vi "Example Write Read Type 2 - StateChanged Callback.vi"(4 "StateChanged":refnum<user-event>, 5 "Event Data":T1, 6 "Control Ref":refnum<k24>, 7 "Event Common Data":T2) -> ()   [LabVIEW 2010]
uses:
  C:/tf/play/labview/Tinkerforge.dll
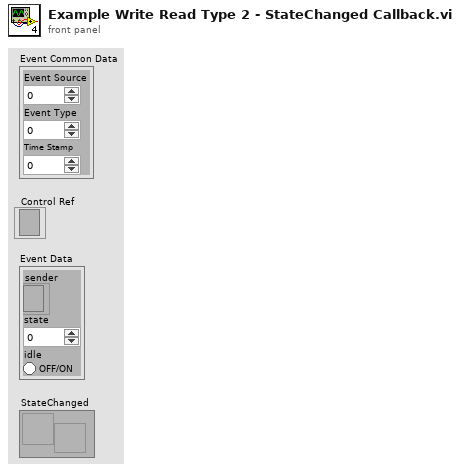
[diagram p1: front panel]
types:
  T1 = cluster{"sender":refnum<k24>, "state":u8, "idle":bool}
  T2 = cluster{"Event Source":i32, "Event Type":u32, "Time Stamp":u32}
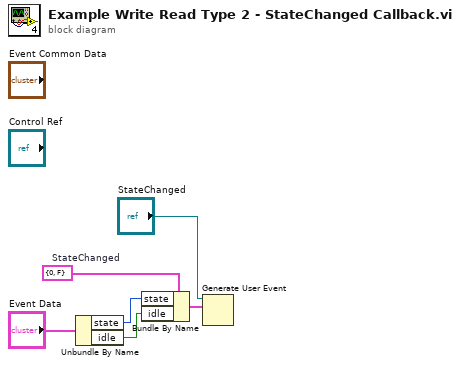
[diagram p0: block diagram]
diagram:
  w5 = cluster{"state":u8, "idle":bool} {"state"=0, "idle"=FALSE}  # StateChanged
  n1 = Unbundle By Name("Event Data") -> ("state"=w4:u8, "idle"=w3:bool)
  n2 = Bundle By Name(cluster=w5, "state"=w4, "idle"=w3) -> (w1:cluster{"state":u8, "idle":bool})
  n3 = Generate User Event(user event="StateChanged", event data cluster=w1) -> ()  [unwired: 1 in, 2 out]
